vi "CS_cRIO_PB_FPGA_DP-MasterProcessData.vi"() -> ()   [LabVIEW 2013]
uses:
  <vilib>/rvi/Emulation/niFpgaSctlEmulationGetInTimedLoop.vi
  <vilib>/rvi/Emulation/niFpgaProcessEmulError.vi
  <vilib>/rvi/Emulation/niFpgaEmulationReportErrorSimple.vi
  <vilib>/rvi/Emulation/niFpgaGetClockAttributes.vi
  <vilib>/rvi/Memory/Memory_Emulation/nirvimemoryEmulation.vi
  <vilib>/rvi/Memory/Memory_Emulation/nirvimemoryFastEmulation.vi
  <vilib>/rvi/DataTransferAndStorage/Container/Common/niFpgaContainerGetUniqueNameForEmu.vi
  <vilib>/rvi/Memory/Memory_Emulation/niFpgaMemoryEmulationCacheClearOnFirstRun.vi
  <vilib>/rvi/Memory/Memory_Emulation/nirvimemoryEmulationManagerCache_MakeExclusive.vi
  <vilib>/rvi/Memory/Memory_Emulation/niFpgaMemoryEmulationValidateCache.vi
  <vilib>/rvi/Memory/Memory_Emulation/nirvimemoryEmulationManagerCache_ReleaseExclusive.vi
  <vilib>/rvi/Memory/Memory_Emulation/nirvimemoryEmulationManagerCache_InsertValue.vi
  <vilib>/Utility/error.llb/Clear Errors.vi
  <vilib>/rvi/Memory/Memory_Emulation/nirvimemoryEmulationManagerCache_SetValue.vi
  <vilib>/rvi/Emulation/niFpgaSctlEmulationResourceMgr.vi
  <vilib>/rvi/Memory/Memory_Emulation/nirvimemoryEmulationManagerCache_GetValue.vi
  <vilib>/rvi/interface/RandomDataEmulation/nirviRandomDataFPGAFIFO.vi
  <vilib>/rvi/interface/RandomDataEmulation/niFpgaRandomDataHandleErrors.vi
  <vilib>/rvi/Emulation/niFpgaCriticalErrorInLSC.vi
  <vilib>/rvi/DataTransferAndStorage/Container/XNode/niFpgaContainer.xnode
  <vilib>/rvi/interface/RandomDataEmulation/nirviRandomDataFpgaReadWriteTemplate.vi
panel:
  out "Zeit seit letztem Aufruf [us]":u32
  in  "zu setzender Zählerwert":u16[](array[numeric])=[0, 0, 0, 0, 0, 0, 0, 0, 0, 0, 0, 0, 0, 0, 0, 0, 0, 0, 0, 0, 0, 0, 0, 0, 0, 0, 0, 0, 0, 0]
  in  "Zähler zurücksetzen":bool[](array[boolean])=[FALSE, FALSE, FALSE, FALSE, FALSE, FALSE, FALSE, FALSE, FALSE, FALSE, FALSE, FALSE, FALSE, FALSE, FALSE, FALSE, FALSE, FALSE, FALSE, FALSE, FALSE, FALSE, FALSE, FALSE, FALSE, FALSE, FALSE, FALSE, FALSE, FALSE]
  in  "Zähler-Einstellung":T1(array[cluster])=[{"Index (Station/Band)"=0, "Station/Band"=enum."Station", "Bitstelle"=0, "Zählrichtung"=enum."Hochzählen"}, {"Index (Station/Band)"=0, "Station/Band"=enum."Station", "Bitstelle"=0, "Zählrichtung"=enum."Hochzählen"}, {"Index (Station/Band)"=0, "Station/Band"=enum."Station", "Bitstelle"=0, "Zählrichtung"=enum."Hochzählen"}, {"Index (Station/Band)"=0, "Station/Band"=enum."Station", "Bitstelle"=0, "Zählrichtung"=enum."Hochzählen"}, {"Index (Station/Band)"=0, "Station/Band"=enum."Station", "Bitstelle"=0, "Zählrichtung"=enum."Hochzählen"}, {"Index (Station/Band)"=0, "Station/Band"=enum."Station", "Bitstelle"=0, "Zählrichtung"=enum."Hochzählen"}, {"Index (Station/Band)"=0, "Station/Band"=enum."Station", "Bitstelle"=0, "Zählrichtung"=enum."Hochzählen"}, {"Index (Station/Band)"=0, "Station/Band"=enum."Station", "Bitstelle"=0, "Zählrichtung"=enum."Hochzählen"}, {"Index (Station/Band)"=0, "Station/Band"=enum."Station", "Bitstelle"=0, "Zählrichtung"=enum."Hochzählen"}, {"Index (Station/Band)"=0, "Station/Band"=enum."Station", "Bitstelle"=0, "Zählrichtung"=enum."Hochzählen"}, {"Index (Station/Band)"=0, "Station/Band"=enum."Station", "Bitstelle"=0, "Zählrichtung"=enum."Hochzählen"}, {"Index (Station/Band)"=0, "Station/Band"=enum."Station", "Bitstelle"=0, "Zählrichtung"=enum."Hochzählen"}, {"Index (Station/Band)"=0, "Station/Band"=enum."Station", "Bitstelle"=0, "Zählrichtung"=enum."Hochzählen"}, {"Index (Station/Band)"=0, "Station/Band"=enum."Station", "Bitstelle"=0, "Zählrichtung"=enum."Hochzählen"}, {"Index (Station/Band)"=0, "Station/Band"=enum."Station", "Bitstelle"=0, "Zählrichtung"=enum."Hochzählen"}, {"Index (Station/Band)"=0, "Station/Band"=enum."Station", "Bitstelle"=0, "Zählrichtung"=enum."Hochzählen"}, {"Index (Station/Band)"=0, "Station/Band"=enum."Station", "Bitstelle"=0, "Zählrichtung"=enum."Hochzählen"}, {"Index (Station/Band)"=0, "Station/Band"=enum."Station", "Bitstelle"=0, "Zählrichtung"=enum."Hochzählen"}, {"Index (Station/Band)"=0, "Station/Band"=enum."Station", "Bitstelle"=0, "Zählrichtung"=enum."Hochzählen"}, {"Index (Station/Band)"=0, "Station/Band"=enum."Station", "Bitstelle"=0, "Zählrichtung"=enum."Hochzählen"}, {"Index (Station/Band)"=0, "Station/Band"=enum."Station", "Bitstelle"=0, "Zählrichtung"=enum."Hochzählen"}, {"Index (Station/Band)"=0, "Station/Band"=enum."Station", "Bitstelle"=0, "Zählrichtung"=enum."Hochzählen"}, {"Index (Station/Band)"=0, "Station/Band"=enum."Station", "Bitstelle"=0, "Zählrichtung"=enum."Hochzählen"}, {"Index (Station/Band)"=0, "Station/Band"=enum."Station", "Bitstelle"=0, "Zählrichtung"=enum."Hochzählen"}, {"Index (Station/Band)"=0, "Station/Band"=enum."Station", "Bitstelle"=0, "Zählrichtung"=enum."Hochzählen"}, {"Index (Station/Band)"=0, "Station/Band"=enum."Station", "Bitstelle"=0, "Zählrichtung"=enum."Hochzählen"}, {"Index (Station/Band)"=0, "Station/Band"=enum."Station", "Bitstelle"=0, "Zählrichtung"=enum."Hochzählen"}, {"Index (Station/Band)"=0, "Station/Band"=enum."Station", "Bitstelle"=0, "Zählrichtung"=enum."Hochzählen"}, {"Index (Station/Band)"=0, "Station/Band"=enum."Station", "Bitstelle"=0, "Zählrichtung"=enum."Hochzählen"}, {"Index (Station/Band)"=0, "Station/Band"=enum."Station", "Bitstelle"=0, "Zählrichtung"=enum."Hochzählen"}]
  out "Zählerwerte":u16[](array[numeric])
  in  "Slave address:":u8 caption="Only for command 0x87\n - Read diagnostic data"
  out "SPI Frame error:":bool
  out "Timed out:":bool caption="Timed out"
  out "Driver RC:":u8 format="%.0x"
  in  "Input length":u16=8 caption="Length"
  in  "Output length":u16=8 caption="Length"
  in  "Delay":u32=10 caption="Delay (µs):"
  out "Status:":u8 format="%.0x"
  in  "Write output data:":u8[](array[numeric])=[0, 0, 0, 0, 0, 0, 0, 0, 0, 0, 0, 0, 0, 0, 0, 0, 0, 0, 0, 0] format="%.0x"
  in  "Stop":bool
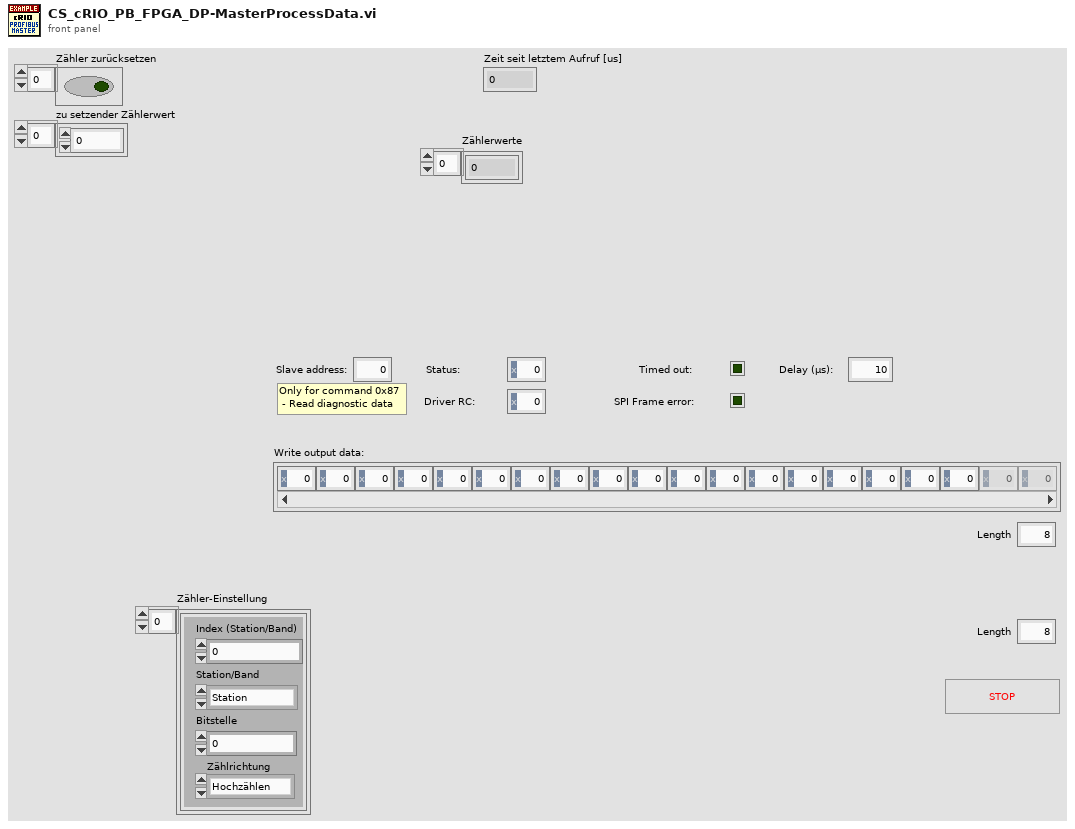
[diagram p1: front panel]
types:
  T1 = cluster{"Index (Station/Band)":u8, "Station/Band":enum16{"Station", "Band"}, "Bitstelle":u8, "Zählrichtung":enum16{"Hochzählen", "Runterzählen"}}[]
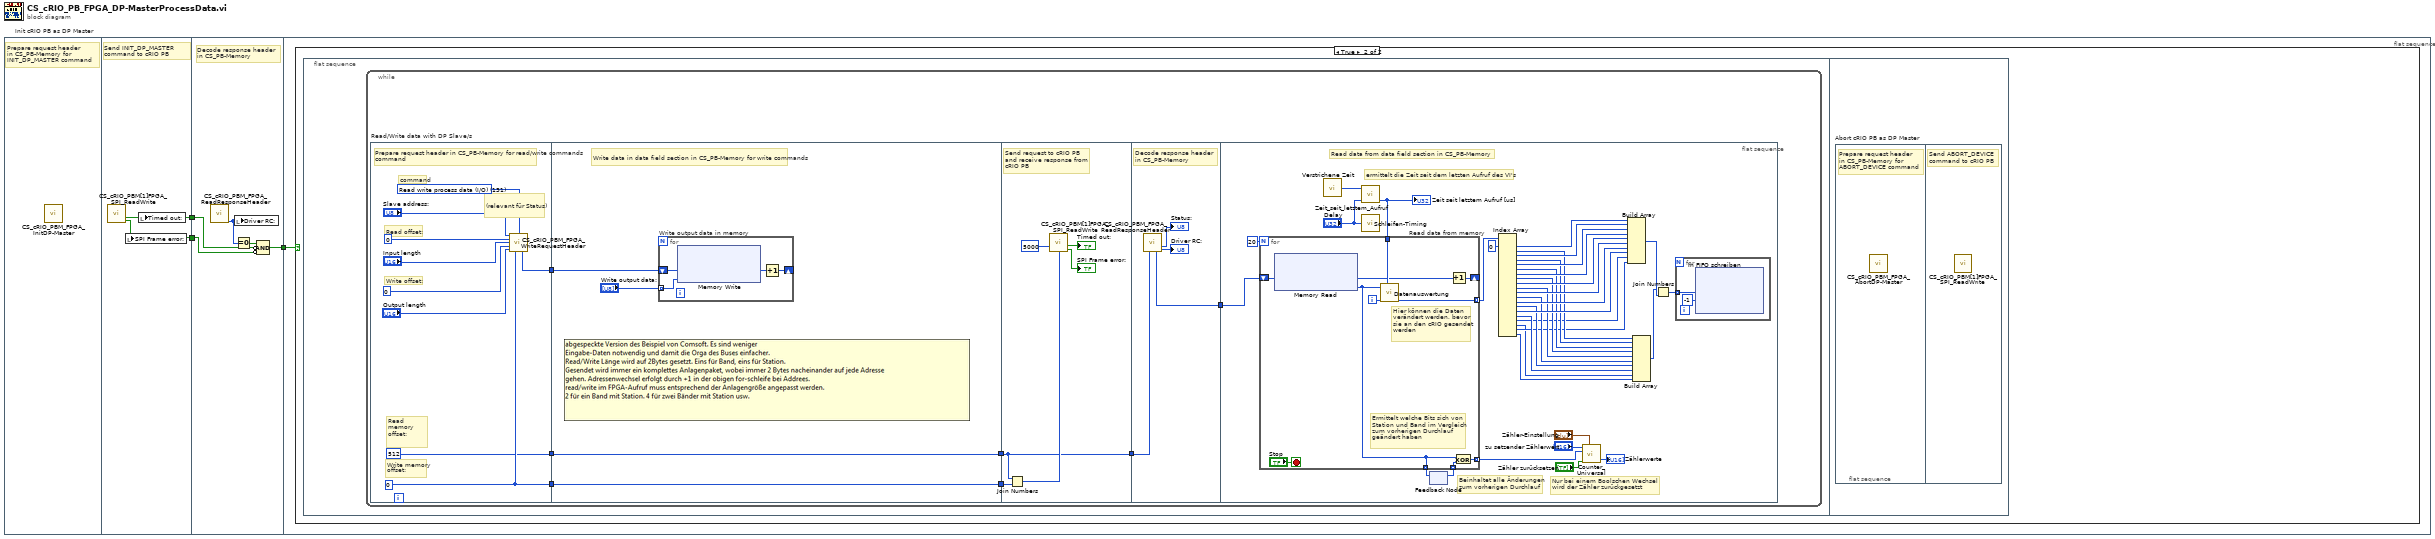
[diagram p0: block diagram]
diagram:
  n1 = flat-sequence "Init cRIO PB as DP Master" {
    tunnel: [w5] -> w3
    tunnel: [w4] -> w2
    tunnel: w3 -> [w9]
    tunnel: w2 -> [w8]
    tunnel: [w6] -> w1
    tunnel: w1 -> [w11]
    frame #0 {
      # "Prepare request header \nin CS_PB-Memory for \nINIT_DP_MASTER command"
      n2 = call <vilib>:"CS_cRIO_PBM_FPGA_InitDP-Master.vi"() -> ()  [unwired: 15 in, 1 out]
    }
    frame #1 {
      # "Send INIT_DP_MASTER\ncommand to cRIO PB"
      n3 = call <vilib>:"CS_cRIO_PBM[1]FPGA_SPI_ReadWrite.vi"() -> ("Timed out"=w5:bool, "Error"=w4:bool)  [unwired: 14 in]
      n4 = local write "SPI Frame error:"(w4) -> ()
      n5 = local write "Timed out:"(w5) -> ()
    }
    frame #2 {
      # "Decode response header \nin CS_PB-Memory"
      n6 = call <vilib>:"CS_cRIO_PBM_FPGA_ReadResponseHeader.vi"() -> ("Driver RC:"=w7:u8)  [unwired: 13 in, 2 out]
      n7 = local write "Driver RC:"(w7) -> ()
      n8 = Equal To 0?(x=w7) -> (x = 0?=w10:bool)
      n9 = Compound Arithmetic op=AND(w10, invert w9, invert w8) -> (w6:bool)
    }
    frame #3 {
      n10 = case shown="True" w11 {
        frame False {
        }
        frame True {
          n11 = flat-sequence {
            frame #0 {
              n12 = while {
                stop <- "Stop" stop-if-true
                n13 = flat-sequence "Read/Write data with DP Slave/s" {
                  tunnel: [w28] -> w18
                  tunnel: [w26] -> w17
                  tunnel: [u16 512 ("Read memory\noffset:")] -> w13
                  tunnel: w18 -> [w31]
                  tunnel: [w30] -> w16
                  tunnel: w17 -> [w30]
                  tunnel: w13 -> [w29]
                  tunnel: [w29] -> w12
                  tunnel: w16 -> [w38]
                  tunnel: [w37] -> w15
                  tunnel: w12 -> [w37]
                  tunnel: w15 -> [w45]
                  tunnel: [w42] -> w14
                  tunnel: w14 -> [w82]
                  frame #0 {
                    w22 = u8 131 items=["Read write process data (I/O)"=131, "Read slave diagnostic data"=135, "Read process status list"=141, "Read process output data"=133, "Read process input offsets"=136, "Read process output offsets"=137, "Read process input length"=138, "Read process output length"=139] ("Read/write command:")
                    w26 = u16 0 ("Write memory\noffset:")
                    # "(relevant für Status)"
                    # "Read offset:"
                    # "command"
                    # "Write offset:"
                    # "Read memory\noffset:"
                    # "Write memory\noffset:"
                    # "Prepare request header in CS_PB-Memory for read/write commands \ncommand"
                    n14 = call <vilib>:"CS_cRIO_PBM_FPGA_WriteRequestHeader.vi"("Address:"="Slave address:", "Command"=w22, "InputOffset:"=u16 0, "InputLength:"="Input length", "OutputOffset:"=u16 0, "OutputLength:"="Output length", "Memory address:"=w26) -> ("Next address:"=w28:u16)  [unwired: 8 in]
                  }
                  frame #1 {
                    # "Write data in data field section in CS_PB-Memory for write commands"
                    n15 = for "Write output data in memory" {
                      shift-right: [w33] -> _
                      shift-left: w31 -> [w34]
                      tunnel: "Write output data:" -> [w35] mode=indexing
                      n16 = xnode ("Memory Write")("Adresse"=w34, "Daten"=w35) -> ()  [unwired: 1 in, 1 out]
                      n17 = Increment(x=w34) -> (x+1=w33:u16)
                    }
                  }
                  frame #2 {
                    # "Send request to cRIO PB\nand receive response from\ncRIO PB"
                    n18 = Join Numbers(hi=w37, lo=w38) -> ((hi.lo)=w39:u32)
                    n19 = call <vilib>:"CS_cRIO_PBM[1]FPGA_SPI_ReadWrite.vi"("Timeout (ms)"=u16 5000, "Memory address:"=w39) -> ("Timed out"=→"Timed out:":bool, "Error"=→"SPI Frame error:":bool)  [unwired: 12 in]
                  }
                  frame #3 {
                    # "Decode response header \nin CS_PB-Memory"
                    n20 = call <vilib>:"CS_cRIO_PBM_FPGA_ReadResponseHeader.vi"("Memory address:"=w45) -> ("Slave status:"=→"Status:":u8, "Next address:"=w42:u16, "Driver RC:"=→"Driver RC:":u8)  [unwired: 12 in]
                  }
                  frame #4 {
                    # "Nur bei einem Boolschen Wechsel \nwird der Zähler zurückgesetzt"
                    # "ermittelt die Zeit seit dem letzten Aufruf des VI's"
                    # "Beinhaltet alle Änderungen\nzum vorherigen Durchlauf"
                    # "Read data from data field section in CS_PB-Memory"
                    n21 = call "Verstrichene Zeit"() -> ("Tick Count(uSec)"=w79:u16)
                    n22 = call "Zeit_seit_letztem_Aufruf.vi"("mittlere Schleifenperiode"="Delay", "Verstrichene Zeit [us]"=w79) -> ("Zeit seit letztem Aufruf [us]"=w78:u32)  [unwired: 3 in]
                    "Zeit seit letztem Aufruf [us]" <- w78
                    n23 = call "Schleifen-Timing"("Count(uSec)"="Delay") -> ()  [unwired: 1 out]
                    n24 = feedback #1() -> (w76:u8[])  [unwired: 1 in]
                    n25 = for "Read data from memory" {
                      N: 20 -> [_]
                      shift-right: [w91] -> _
                      shift-left: w82 -> [w86]
                      tunnel: w78 -> [w90]
                      tunnel: [w89] -> w75 mode=indexing
                      tunnel: [w87] -> w77 mode=indexing
                      tunnel: w76 -> [w88] mode=indexing
                      tunnel: [w85] -> w70 mode=indexing
                      i -> [w92]
                      # "Ermittelt welche Bits sich von\nStation und Band im Vergleich\nzum vorherigen Durchlauf \ngeändert haben"
                      # "Hier können die Daten\nverändert werden, bevor\nsie an den cRIO gesendet\nwerden"
                      n26 = xnode ("Memory Read")("Adresse"=w86) -> ("Daten"=w87:u8)  [unwired: 1 in, 1 out]
                      n27 = call "Datenauswertung.vi"("Zeit seit dem letzten Aufruf"=w90, "Iterationszähler"=w92, "Daten aus FPGA-Speicher"=w87) -> ("Daten für FIFO"=w85:u8)  [unwired: 8 in]
                      n28 = Increment(x=w86) -> (x+1=w91:u16)
                      n29 = Exclusive Or(1:w88, 2:w87) -> (0:w89:u8)
                    }
                    n30 = feedback-in #1(w77) -> ()
                    n31 = Index Array(array=w70, index #1=0 ("Index")) -> (element #1=w68:u8, element #2=w60:u8, element #3=w67:u8, element #4=w59:u8, element #5=w66:u8, element #6=w58:u8, element #7=w65:u8, element #8=w57:u8, element #9=w64:u8, element #10=w56:u8, element #11=w63:u8, element #12=w55:u8, element #13=w62:u8, element #14=w53:u8, element #15=w61:u8, element #16=w54:u8, element #17=w49:u8, element #18=w46:u8, element #19=w48:u8, element #20=w47:u8)  [unwired: 19 in]
                    n32 = call "Counter_Universal.vi"("zu setzender Zählerwert"="zu setzender Zählerwert", "Änderungen der Station-/Banddaten"=w75, "Zähler zurücksetzen"="Zähler zurücksetzen", "Zähler-Einstellung"="Zähler-Einstellung") -> ("Counter"=→"Zählerwerte":u16[])  [unwired: 3 in]
                    n33 = Build Array(w68, w67, w66, w65, w64, w63, w62, w61, w49, w48) -> (w52:u8[])
                    n34 = Build Array(w60, w59, w58, w57, w56, w55, w53, w54, w46, w47) -> (w51:u8[])
                    n35 = Join Numbers(hi=w51, lo=w52) -> ((hi.lo)=w50:u16[])
                    n36 = for {
                      tunnel: w50 -> [w84] mode=indexing
                      n37 = xnode ("In FIFO schreiben")("Element"=w84, "Timeout"=-1) -> ()  [unwired: 1 in, 2 out]
                    }
                  }
                }
              }
            }
            frame #1 {
              n38 = flat-sequence "Abort cRIO PB as DP Master" {
                frame #0 {
                  # "Prepare request header \nin CS_PB-Memory for \nABORT_DEVICE command"
                  n39 = call <vilib>:"CS_cRIO_PBM_FPGA_AbortDP-Master.vi"() -> ()  [unwired: 15 in, 1 out]
                }
                frame #1 {
                  # "Send ABORT_DEVICE\ncommand to cRIO PB"
                  n40 = call <vilib>:"CS_cRIO_PBM[1]FPGA_SPI_ReadWrite.vi"() -> ()  [unwired: 14 in, 2 out]
                }
              }
            }
          }
        }
      }
    }
  }
